vi "fgv_params_save-load_reg.vi"(7 "cmd":T1(ring), 8 "error in":errorcluster, 11 "file name":string) -> (0 "error out":errorcluster, 3 "open cancelled":bool caption="취소됨")   [LabVIEW 2019]
uses:
  Global_params_reg.vi
  <vilib>/Utility/xml.llb/Write to XML File(string).vi
  <vilib>/Utility/xml.llb/Read From XML File(string).vi
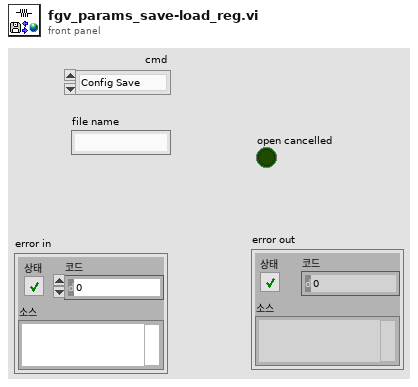
[diagram p1: front panel]
types:
  T1 = enum16{"Config Save", "Config Load", "LastRUN Save", "LastRUN Load"}
  T2 = typedef "config_aging.ctl" = cluster{"CapTest Config":T3, "TestName":string, "Result path":path, "파일 생성 주기[N]":dbl, "CapTest Specs":T4}
  T3 = typedef "Setting_reg.ctl" = cluster{"제어 전압[V]":dbl, "출력전압[V]":dbl, "전류[A]":dbl, "출력전류[A]":dbl, "ON[초]":dbl, "OFF[초]":dbl, "시험횟수[N]":u32, "Irms 허용치 from ":dbl, "Irms 허용치 to":dbl, "Ch selection":cluster{"ch 1":bool, "ch 2":bool, "ch 3":bool, "ch 4":bool, "ch 5":bool, "ch 6":bool}, "AO Delay ms":u32}
  T4 = typedef "공통_내구 진단모드.ctl" = cluster{"제어단 단선[A]":dbl, "제어단 단락[A]":dbl, "제어단 특성변화[A] From":dbl, "제어단 특성변화[A] to":dbl, "출력단 단선[A]":dbl, "출력단 단락[A]":dbl, "출력단 특성변화[A] From":dbl, "출력단 특성변화[A] to":dbl, "부하전압[+/-%] ":dbl, "온도[degree]":dbl}
  T5 = typedef "DL950_config.ctl" = cluster{"Timeout":u32, "Time Div":i32, "Acq Mode":i32, "Record Len":i32, "Record Num":i32, "Start Point":i64, "End Poin":i64, "Visa":refnum<visa-resource-name>, "Config Voltage":cluster{"Enable":bool, "Ch":u16, "V Div":i32, "Coupling":i32, "Probe":i32, "Act.Items":bool, "items":i32[]}[], "Trigger on":bool, "Trigger Level":dbl, "Reset":bool, "Config Temp":cluster{"Channel":u16, "Burn Out":bool, " Type ":i32}[], "Trigger Mode":i32, "Trigger Position":dbl, "Trigger Slope":i32, "Trigger Source ":i32, "Start Point (-5.00)":dbl, "End Point (5.00)":dbl}
  T6 = typedef "BP4610_config.ctl" = cluster{"VISA":refnum<visa-resource-name>, "Limit-BP":cluster{"Set":enum16{"Current", "Voltage"}, "Voltage+[V]":dbl, "Current+[A]":dbl, "Voltage-[V]":dbl, "Current-[A]":dbl}, "SET BP":cluster{"Set":enum16{"Current", "Voltage", "FREQ/WAVE"}, "Operation mode":u16, "Voltage[Vp-p]":dbl, "Current[Ap-p]":dbl, "Voltage[V]":dbl, "Current[A]":dbl, "Frequency[Hz]":dbl, "Waveform":enum16{"Sine", "Square", "ARB 1", "ARB 2", "ARB 3", "ARB 4", "ARB 5", "ARB 6", "ARB 7", "ARB 8", "ARB 9", "ARB 10", "ARB 11", "ARB 12", "ARB 13", "ARB 14", "ARB 15", "ARB 16"}}}
  T7 = typedef "DSP_config.ctl" = cluster{"Port":refnum<visa-resource-name>, "OVP Level":dbl, "OCP Level":dbl, "Current":dbl, "Voltage":dbl}
  T8 = typedef "Set_NIAI.ctl" = cluster{"input terminal":i32, "minimum value":dbl, "maximum value":dbl, "number of samples":i32, "rate":dbl, "sample mode":i32, "physical channels":tag}
  T9 = typedef "cDAQ-9269 Config.ctl" = cluster{"Ch":tag, "Max V":dbl, "Min V":dbl, " Rate":dbl, "N pts":i32, "sample mode":i32}
  T10 = typedef "Set_AO_Wave-config.ctl" = cluster{"offset":dbl, "Number of Samples":i32, "duty cycle (%)":dbl, "Sample Rate":dbl, "Waveform":cluster{"Frequency":dbl, "Amplitude":dbl, "Waveform Type":enum16{"Sine Wave", "Triangle Wave", "Square Wave", "Sawtooth Wave"}}}
  T11 = cluster{"Params":T2, "DL950_config":T5, "BP4610 Config":T6, "DSP1950 Config":T7, "DMM 2470 Config":cluster{"Source Mode":enum16{"Voltage", "Current"}, "Source Limit Level":dbl, "Source Level":dbl, "Output_2470":bool}, "cDAQ-9221 Config":T8, "cDAQ-9467 Config":tag, "cDAQ-9269 AO Config":T9, "AO_Wave-config":T10}
  T12 = enum16{"open", "replace", "create", "open or create", "replace or create", "replace or create with confirmation"}
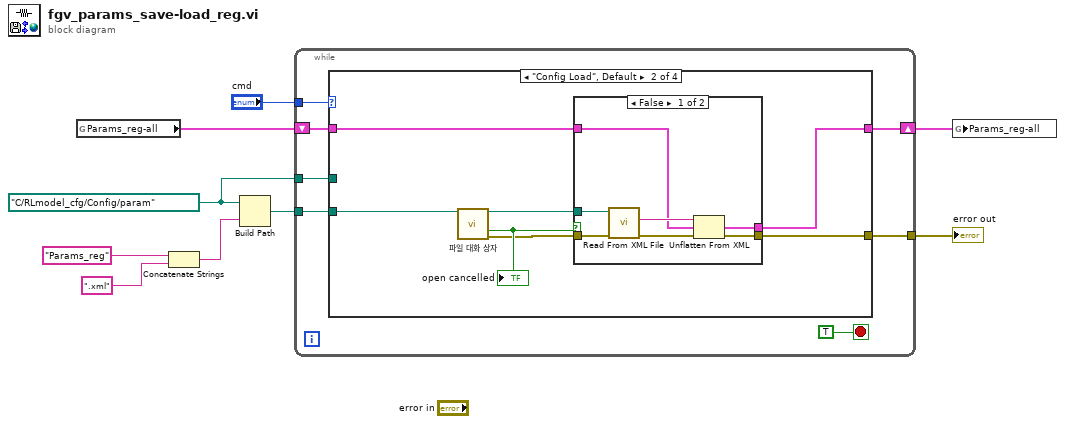
[diagram p0: block diagram]
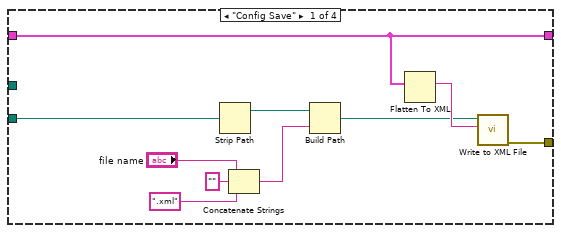
[diagram p2: hidden frame]
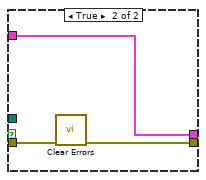
[diagram p3: hidden frame]
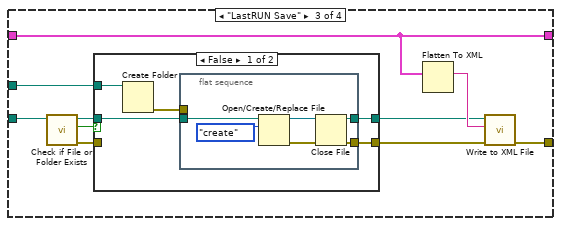
[diagram p4: hidden frame]
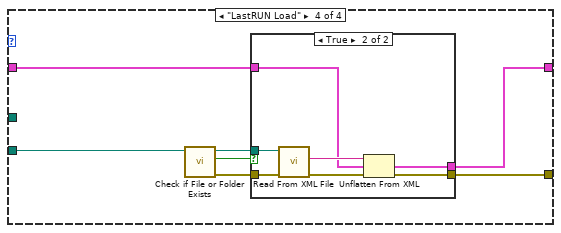
[diagram p6: hidden frame]
diagram:
  w8 = path "C:/RLmodel_cfg/Config/param" ("XML File Path")
  n1 = global read "Global_params_reg.vi" "Params_reg-all"() -> (w2:T11)
  n2 = Concatenate Strings("Params_reg" ("string"), ".xml" ("string")) -> (w4:string)
  n3 = Build Path(base path=w8, name or relative path=w4) -> (appended path=w9:path)
  n4 = while {
    tunnel: [w16] -> w7
    tunnel: "cmd" -> [w15]
    tunnel: w9 -> [w13]
    shift-right: [w12] -> w1
    shift-left: w2 -> [w14]
    tunnel: w8 -> [w10]
    stop <- TRUE stop-if-true
    n5 = case shown="\"Config Load\", Default" w15 {
      tunnel: w14 -> [w21 w30 w47 w73]
      tunnel: w13 -> [w24 w33 w46 w67]
      tunnel: [w25 w28 w48 w71] -> w16
      tunnel: [w21 w27 w47 w72] -> w12
      tunnel: w10 -> [_ _ w44 _]
      frame "Config Save" {
        n6 = Strip Path(path=w24) -> (stripped path=w23:path)  [unwired: 1 out]
        n7 = Concatenate Strings("file name", "" ("문자열"), ".xml" ("문자열")) -> (w22:string)
        n8 = Build Path(base path=w23, name or relative path=w22) -> (appended path=w18:path)
        n9 = Flatten To XML(anything=w21) -> (xml string=w26:string)
        n10 = call-poly <vilib>:"Write to XML File.vi"("XML Input"=w26, "XML File Path"=w18) -> ("error out"=w25:errorcluster)  [unwired: 7 in, 2 out]
      }
      frame "Config Load", Default {
        n11 = call "파일 대화 상자"("start path"=w33) -> ("selected path"=w31:path, "cancelled"=w32:bool, "error out"=w29:errorcluster)  [unwired: 11 in, 1 out]
        "open cancelled" <- w32
        n12 = case shown="False" w32 {
          tunnel: w31 -> [w39 _]
          tunnel: w30 -> [w38 w43]
          tunnel: [w37 w43] -> w27
          tunnel: w29 -> [w35 w42]
          tunnel: [w34 w41] -> w28
          frame False {
            n13 = call-poly <vilib>:"Read From XML File.vi"("error in (no error)"=w35, "XML File Path"=w39) -> ("error out"=w36:errorcluster, "XML Elements"=w40:string)  [unwired: 7 in, 1 out]
            n14 = Unflatten From XML(xml string=w40, type=w38, error in (no error)=w36) -> (value=w37:T11, error out=w34:errorcluster)
          }
          frame True {
            n15 = call <vilib>:"Clear Errors.vi"("error in (no error)"=w42) -> ("error out"=w41:errorcluster)  [unwired: 5 in, 1 out]
          }
        }
      }
      frame "LastRUN Save" {
        n16 = call <vilib>:"Check if File or Folder Exists.vi"("path"=w46) -> ("error out"=w52:errorcluster, "file or folder exists?"=w50:bool, "dup path"=w51:path)  [unwired: 8 in]
        n17 = case shown="False" w50 {
          tunnel: w52 -> [_ w66]
          tunnel: w51 -> [w58 w65]
          tunnel: [w56 w66] -> w49
          tunnel: [w57 w65] -> w45
          tunnel: w44 -> [w55 _]
          frame False {
            n18 = Create Folder(path (use dialog)=w55) -> (error out=w54:errorcluster)  [unwired: 2 in, 2 out]
            n19 = flat-sequence {
              tunnel: w58 -> [w64]
              tunnel: [w60] -> w57
              tunnel: [w59] -> w56
              tunnel: w54 -> [_]
              frame #0 {
                n20 = Open/Create/Replace File(file path (use dialog)=w64, operation (0:open)=T12."create" ("동작(0:open)")) -> (refnum out=w61:refnum<file>, error out=w62:errorcluster)  [unwired: 4 in, 1 out]
                n21 = Close File(refnum=w61, error in=w62) -> (path=w60:path, error out=w59:errorcluster)
              }
            }
          }
          frame True {
          }
        }
        n22 = Flatten To XML(anything=w47) -> (xml string=w53:string)
        n23 = call-poly <vilib>:"Write to XML File.vi"("error in (no error)"=w49, "XML Input"=w53, "XML File Path"=w45) -> ("error out"=w48:errorcluster)  [unwired: 6 in, 2 out]
      }
      frame "LastRUN Load" {
        n24 = call <vilib>:"Check if File or Folder Exists.vi"("path"=w67) -> ("error out"=w68:errorcluster, "file or folder exists?"=w69:bool, "dup path"=w70:path)  [unwired: 8 in]
        n25 = case shown="True" w69 {
          tunnel: w73 -> [_ w80]
          tunnel: [_ w79] -> w72
          tunnel: [w74 w77] -> w71
          tunnel: w70 -> [_ w76]
          tunnel: w68 -> [w74 w75]
          frame False {
          }
          frame True {
            n26 = call-poly <vilib>:"Read From XML File.vi"("error in (no error)"=w75, "XML File Path"=w76) -> ("error out"=w78:errorcluster, "XML Elements"=w81:string)  [unwired: 7 in, 1 out]
            n27 = Unflatten From XML(xml string=w81, type=w80, error in (no error)=w78) -> (value=w79:T11, error out=w77:errorcluster)
          }
        }
      }
    }
  }
  "error out" <- w7
  n28 = global write "Global_params_reg.vi" "Params_reg-all"(w1) -> ()
